vi "thorlabs_get_status_bits.vi"(8 "error in (no error)":errorcluster, 10 "channel":i16, 11 "thorlabs_kinesis in":refnum<class "thorlabs_kinesis.lvclass">) -> (0 "error out":errorcluster, 2 "status_bits":i32, 3 "thorlabs_kinesis out":refnum<class "thorlabs_kinesis.lvclass">)   [LabVIEW 2015, in "thorlabs_kinesis.lvclass"]
uses:
  thorlabs_kinesis.lvclass
  thorlabs_kinesis.lvclass/thorlabs_kinesis.ctl
  thorlabs_drivers/Thorlabs.MotionControl.Benchtop.Piezo.dll
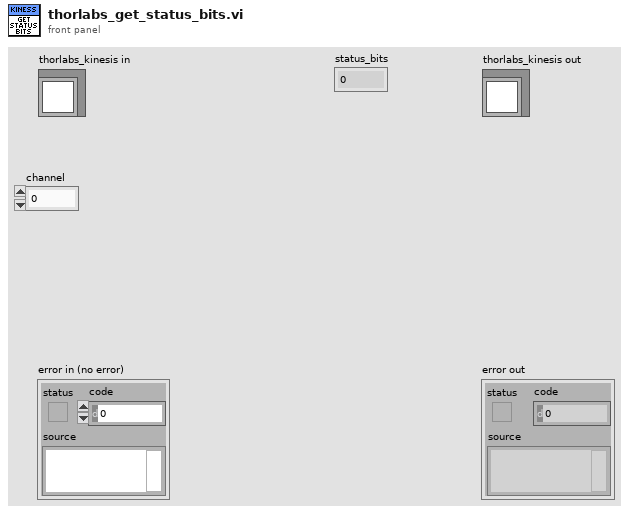
[diagram p1: front panel]
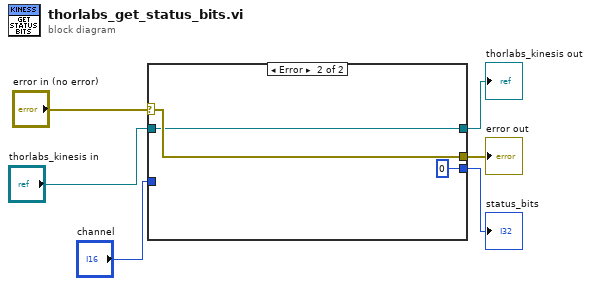
[diagram p0: block diagram]
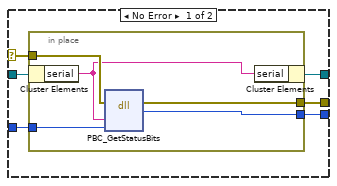
[diagram p2: hidden frame]
diagram:
  n1 = case shown="Error" "error in (no error)" {
    selector: "error in (no error)" -> [w11 w20]
    tunnel: [w10 w20] -> w5
    tunnel: [w8 w19] -> w3
    tunnel: "thorlabs_kinesis in" -> [w12 w19]
    tunnel: "channel" -> [w9 _]
    tunnel: [w7 0 ("return type")] -> w1
    frame No Error {
      n2 = in-place {
        in-place-border: w11 -> [w17]
        in-place-border: [w16] -> w10
        in-place-border: w9 -> [w15]
        in-place-border: [w13] -> w7
        n3 = in-place-cluster #1(w12) -> ("serial"=w14:string)
        n4 = dll-call lib="C:/Users/bspoka/Documents/LabVIEW Data/lview_180307/Stage Class/Thorlabs Kinesis/thorlabs_drivers/Thorlabs.MotionControl.Benchtop.Piezo.dll" fn="PBC_GetStatusBits" label="PBC_get_status_bits"(error in=w17, "serial"=w14, "channel"=w15) -> (error out=w16:errorcluster, "return type"=w13:i32)  [unwired: 4 in, 1 out]
        n5 = in-place-cluster #1("serial"=w14) -> (w8:refnum<class "thorlabs_kinesis.lvclass">)
      }
    }
    frame Error {
    }
  }
  "error out" <- w5
  "thorlabs_kinesis out" <- w3
  "status_bits" <- w1
